vi "Twist_Angle_2.vi"(11 "Xt":dbl format="%#_13g") -> (3 "TA":dbl)   [LabVIEW 2019, in "Algorithm.lvclass"]
uses:
  FrameworkOverrides/Algorithm.lvclass
panel:
  out "C":dbl
  out "B":dbl
  out "A":dbl
  in  "Theta":dbl=18.5
  in  "T":dbl=0.35 format="%#_13g"
  in  "W":dbl=1.8 format="%#_13g"
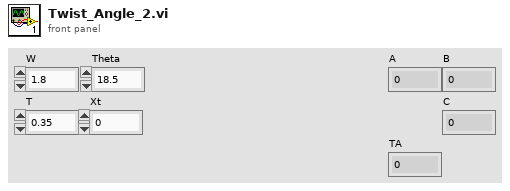
[diagram p1: front panel]
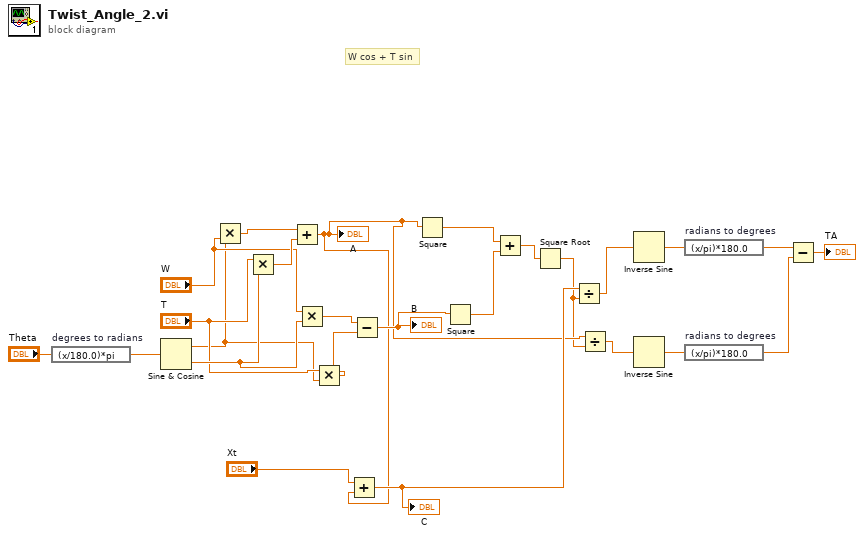
[diagram p0: block diagram]
diagram:
  # "W cos + T sin"
  n1 = expression code="(x/180.0)*pi" "degrees to radians"("Theta") -> (w19:dbl)
  n2 = Sine & Cosine(0:w19) -> (1:w12:dbl, 2:w15:dbl)
  n3 = Multiply(x=w12, y="W") -> (x*y=w18:dbl)
  n4 = Multiply(x="T", y=w15) -> (x*y=w17:dbl)
  n5 = Add(x=w18, y=w17) -> (x+y=w4:dbl)
  "A" <- w4
  n6 = Multiply(x="W", y=w15) -> (x*y=w14:dbl)
  n7 = Multiply(x="T", y=w12) -> (x*y=w11:dbl)
  n8 = Add(x="Xt", y=w4) -> (x+y=w5:dbl)
  "C" <- w5
  n9 = Subtract(x=w14, y=w11) -> (x-y=w9:dbl)
  "B" <- w9
  n10 = Square(x=w4) -> (x^2=w8:dbl)
  n11 = Square(x=w9) -> (x^2=w7:dbl)
  n12 = Add(x=w8, y=w7) -> (x+y=w6:dbl)
  n13 = Square Root(x=w6) -> (sqrt(x)=w3:dbl)
  n14 = Divide(x=w5, y=w3) -> (x/y=w2:dbl)
  n15 = Divide(x=w4, y=w3) -> (x/y=w1:dbl)
  n16 = Inverse Sine(1:w2) -> (0:w25:dbl)
  n17 = Inverse Sine(1:w1) -> (0:w24:dbl)
  n18 = expression code="(x/pi)*180.0" "radians to degrees"(w25) -> (w23:dbl)
  n19 = expression code="(x/pi)*180.0" "radians to degrees"(w24) -> (w22:dbl)
  n20 = Subtract(x=w23, y=w22) -> (x-y=→"TA":dbl)
